vi "PSPOP_Register.vi"(4 "Col (unwired = all columns)":i32=-2, 5 "Name":string, 6 "Row (unwired = all rows)":i32=-2, 7 "Tag (none)":string, 8 "error in (no error)":errorcluster, 9 "Parameters":T1={"Prop Type"=enum."String", "Initial Value"=variant, "Caption Strings"=[], "Ring Strings"=[], "Cell Rect"={"left"=0, "top"=0, "right"=0, "bottom"=0}, "Mouse Coords"={"x"=0, "y"=0}, "Call Data"=variant, "Ring Values"=[], "Browse Options"={"Prompt"="", "Match Pattern"="", "Mode"=enum."existing file", "Start Path"=path "", "Pattern Label"="", "Button Text"=""}, "Combo Box"={"Allow Undefined Strings"=FALSE}}, 11 "Ctl Refnum":refnum<vi>) -> (0 "error out":errorcluster, 3 "dup ref out":refnum<vi>)   [LabVIEW 2016]
uses:
  Private/Ctrls/POP_Popup Call Parameters.ctl
  Private/Ctrls/POP_Data Type.ctl
  <vilib>/Utility/miscctls.llb/LVBrowseOptionsTypeDef.ctl
  Private/Ctrls/POP_Popup Operation.ctl
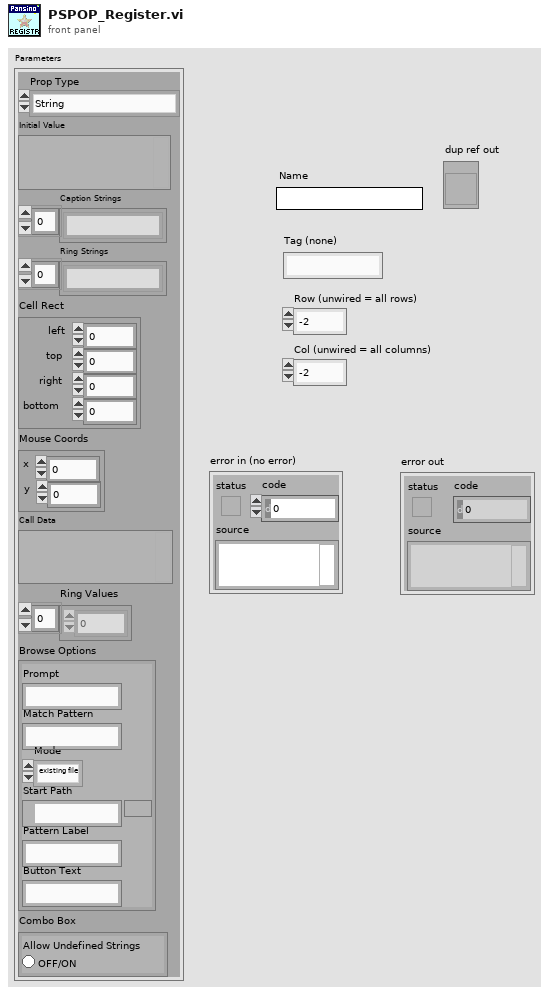
[diagram p1: front panel]
types:
  T1 = typedef "POP_Popup Call Parameters.ctl" = cluster{"Prop Type":T2, "Initial Value":variant, "Caption Strings":string[], "Ring Strings":string[], "Cell Rect":cluster{"left":i16, "top":i16, "right":i16, "bottom":i16}, "Mouse Coords":cluster{"x":i16, "y":i16}, "Call Data":variant, "Ring Values":ext[], "Browse Options":T3, "Combo Box":cluster{"Allow Undefined Strings":bool}}
  T2 = typedef "POP_Data Type.ctl" = enum16{"NO POPUP", "Unkown", "String", "Integer", "Float", "Color", "Boolean", "Ring", "Captioned String", "Captioned Integer", "Button Color", "2 Int Cluster", "4 Int Cluster", "6-Dbl Cluster", "Path", "Combox", "Time", "ShotCut String"}
  T3 = typedef "LVBrowseOptionsTypeDef.ctl" = cluster{"Prompt":string, "Match Pattern":string, "Mode":enum32{"existing file", "new file", "new or existing file", "existing dir", "new dir", "new or existing dir", "existing file (use LLBs)", "new file (use LLBs)", "new or existing file (use LLBs)", "new or existing file or directory (use LLBs)", "existing dir (use LLBs)", "new dir (use LLBs)", "new or existing dir (use LLBs)", "existing file or dir", "new file or dir", "new or existing file or dir", "existing file or dir (use LLBs)", "new file or dir (use LLBs)"}, "Start Path":path, "Pattern Label":string, "Button Text":string}
  T4 = typedef "POP_Popup Operation.ctl" = enum16{"Show", "Initialize", "Close", "Popup Done", "Register a Location's Type", "Retrieve Location's Type"}
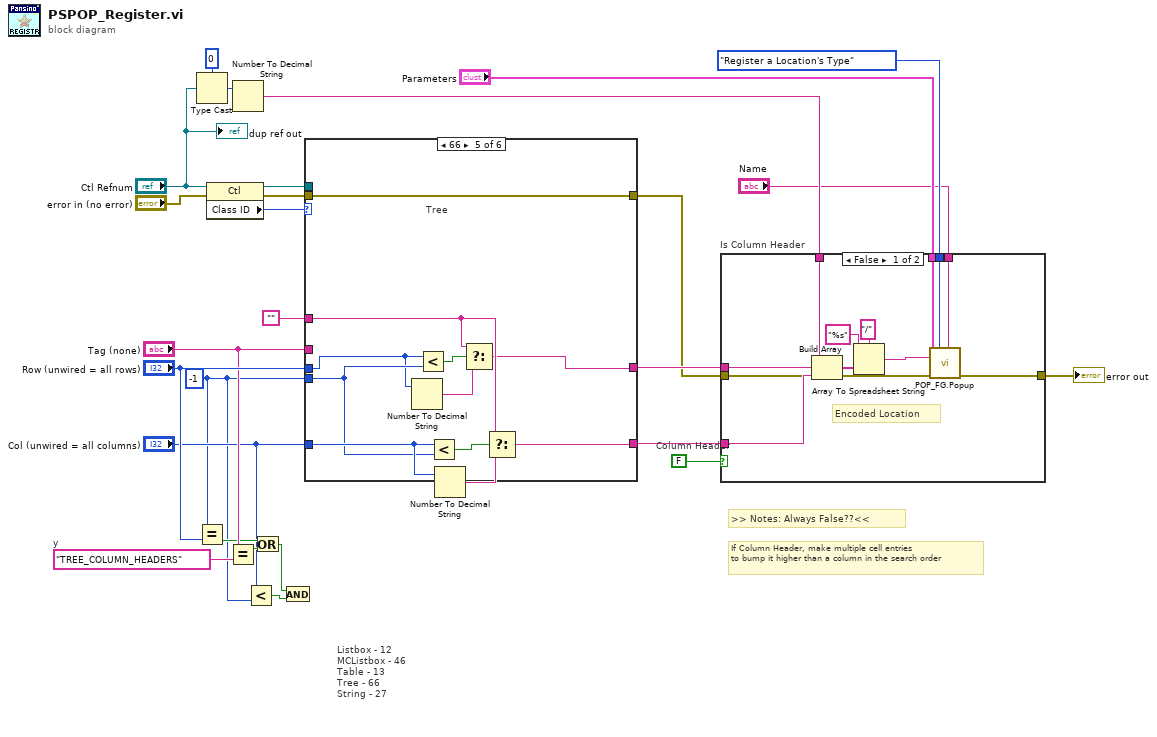
[diagram p0: block diagram]
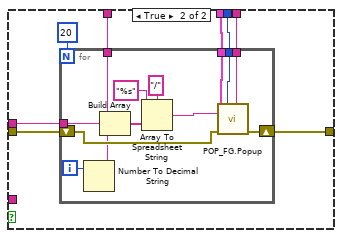
[diagram p2: hidden frame]
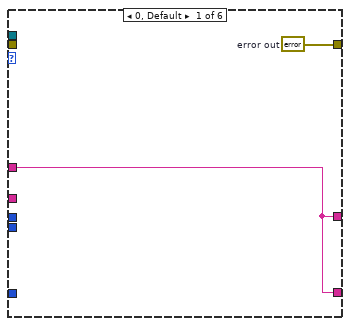
[diagram p3: hidden frame]
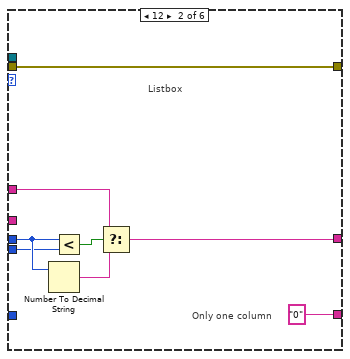
[diagram p4: hidden frame]
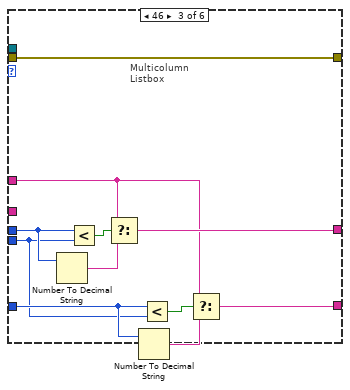
[diagram p5: hidden frame]
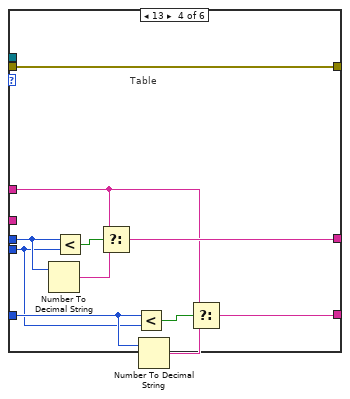
[diagram p6: hidden frame]
diagram:
  w13 = "TREE_COLUMN_HEADERS"  # y
  w5 = -1 ("y")
  # ">> Notes: Always False??<<"
  # "If Column Header, make multiple cell entries\nto bump it higher than a column in the search order"
  # "Column Header"
  # "Listbox - 12\nMCListbox - 46\nTable - 13\nTree - 66\nString - 27"
  n1 = Type Cast(type=0, x="Ctl Refnum") -> (*(type *) &x=w23:i32)
  n2 = Equal?(x=w5, y="Row (unwired = all rows)") -> (x = y?=w11:bool)
  n3 = property class="Ctl"(reference="Ctl Refnum", error in="error in (no error)") -> (reference out=w25:refnum<vi>, error out=w17:errorcluster, "Class ID"=w26:u32)
  n4 = Equal?(x="Tag (none)", y=w13) -> (x = y?=w12:bool)
  n5 = Number To Decimal String(number=w23) -> (decimal integer string=w22:string)  [unwired: 1 in]
  n6 = Less?(x="Col (unwired = all columns)", y=w5) -> (x < y?=w4:bool)
  n7 = Or(x=w11, y=w12) -> (x .or. y?=w3:bool)
  n8 = And(x=w3, y=w4) -> ()  [unwired: 1 out]
  n9 = case shown="66" w26 {
    tunnel: w25 -> [_ _ _ _ _ _]
    tunnel: "Tag (none)" -> [_ _ _ _ _ _]
    tunnel: "Row (unwired = all rows)" -> [_ w31 w40 w52 w61 _]
    tunnel: "Col (unwired = all columns)" -> [_ _ w39 w50 w66 _]
    tunnel: "" -> [w28 w35 w43 w54 w60 w71]
    tunnel: [w28 w34 w46 w57 w59 w71] -> w20
    tunnel: [w28 "0" w44 w55 w68 w71] -> w19
    tunnel: w17 -> [_ w32 w42 w53 w67 w70]
    tunnel: [w27 w32 w42 w53 w67 w70] -> w7
    tunnel: w5 -> [_ w30 w37 w49 w62 _]
    frame 0, Default {
      w27 = errorcluster {"status"=TRUE, "code"=1, "source"="Invalid Control Type"}  # error out
    }
    frame 12 {
      # "Only one column"
      # "Listbox"
      n10 = Number To Decimal String(number=w31) -> (decimal integer string=w36:string)  [unwired: 1 in]
      n11 = Less?(x=w31, y=w30) -> (x < y?=w29:bool)
      n12 = Select(t=w35, s=w29, f=w36) -> (s? t:f=w34:string)
    }
    frame 46 {
      # "Multicolumn\nListbox"
      n13 = Number To Decimal String(number=w40) -> (decimal integer string=w47:string)  [unwired: 1 in]
      n14 = Less?(x=w40, y=w37) -> (x < y?=w41:bool)
      n15 = Select(t=w43, s=w41, f=w47) -> (s? t:f=w46:string)
      n16 = Number To Decimal String(number=w39) -> (decimal integer string=w45:string)  [unwired: 1 in]
      n17 = Less?(x=w39, y=w37) -> (x < y?=w38:bool)
      n18 = Select(t=w43, s=w38, f=w45) -> (s? t:f=w44:string)
    }
    frame 13 {
      # "Table"
      n19 = Number To Decimal String(number=w52) -> (decimal integer string=w58:string)  [unwired: 1 in]
      n20 = Less?(x=w52, y=w49) -> (x < y?=w51:bool)
      n21 = Select(t=w54, s=w51, f=w58) -> (s? t:f=w57:string)
      n22 = Less?(x=w50, y=w49) -> (x < y?=w48:bool)
      n23 = Number To Decimal String(number=w50) -> (decimal integer string=w56:string)  [unwired: 1 in]
      n24 = Select(t=w54, s=w48, f=w56) -> (s? t:f=w55:string)
    }
    frame 66 {
      # "Tree"
      n25 = Number To Decimal String(number=w61) -> (decimal integer string=w64:string)  [unwired: 1 in]
      n26 = Less?(x=w61, y=w62) -> (x < y?=w63:bool)
      n27 = Less?(x=w66, y=w62) -> (x < y?=w65:bool)
      n28 = Number To Decimal String(number=w66) -> (decimal integer string=w69:string)  [unwired: 1 in]
      n29 = Select(t=w60, s=w63, f=w64) -> (s? t:f=w59:string)
      n30 = Select(t=w60, s=w65, f=w69) -> (s? t:f=w68:string)
    }
    frame 27 {
      # "String"
    }
  }
  n31 = case "Is Column Header" shown="False" FALSE {
    tunnel: w22 -> [w80 w91]
    tunnel: w20 -> [w79 w90]
    tunnel: w19 -> [w78 _]
    tunnel: [w76 w89] -> w10
    tunnel: "Parameters" -> [w75 w87]
    tunnel: POP_Popup_Operation."Register a Location's Type" ("Popup Operation") -> [w74 w88]
    tunnel: w7 -> [w73 w86]
    tunnel: "Name" -> [w72 w84]
    frame False {
      # "Encoded Location"
      n32 = Build Array(w80, w79, w78) -> (w83:string[])
      n33 = Array To Spreadsheet String(delimiter (Tab)="/", array=w83, 3:"%s" ("format string")) -> (spreadsheet string=w77:string)
      n34 = call "POP_FG.Popup.vi"("Popup Parameters"=w75, "Popup Operation"=w74, "Name"=w72, "Encoded Location"=w77, "Error In"=w73) -> ("Error Out"=w76:errorcluster)  [unwired: 7 in, 3 out]
    }
    frame True {
      n35 = for {
        N: 20 -> [_]
        tunnel: w91 -> [w101]
        tunnel: w90 -> [w100]
        tunnel: w88 -> [w97]
        tunnel: w87 -> [w96]
        shift-right: [w98] -> w89
        shift-left: w86 -> [w95]
        tunnel: w84 -> [w92]
        i -> [w94]
        n36 = Number To Decimal String(number=w94) -> (decimal integer string=w93:string)  [unwired: 1 in]
        n37 = Build Array(w101, w100, w93) -> (w104:string[])
        n38 = Array To Spreadsheet String(delimiter (Tab)="/", array=w104, 3:"%s" ("format string")) -> (spreadsheet string=w99:string)
        n39 = call "POP_FG.Popup.vi"("Popup Parameters"=w96, "Popup Operation"=w97, "Name"=w92, "Encoded Location"=w99, "Error In"=w95) -> ("Error Out"=w98:errorcluster)  [unwired: 7 in, 3 out]
      }
    }
  }
  "error out" <- w10
  "dup ref out" <- "Ctl Refnum"
